vi "CloseConnection.vi"(8 "error in (no error)":errorcluster, 11 "TCP Connection in":refnum<class "TCP Connection.lvclass">) -> (0 "error out":errorcluster, 3 "TCP Connection out":refnum<class "TCP Connection.lvclass">)   [LabVIEW 2011, in "TCP Connection.lvclass"]
doc: "Close a TCP connection.\n\nAuthor: Jared Kirschner"
uses:
  TCP Connection.lvclass
  TCP Connection.lvclass/TCP Connection.ctl
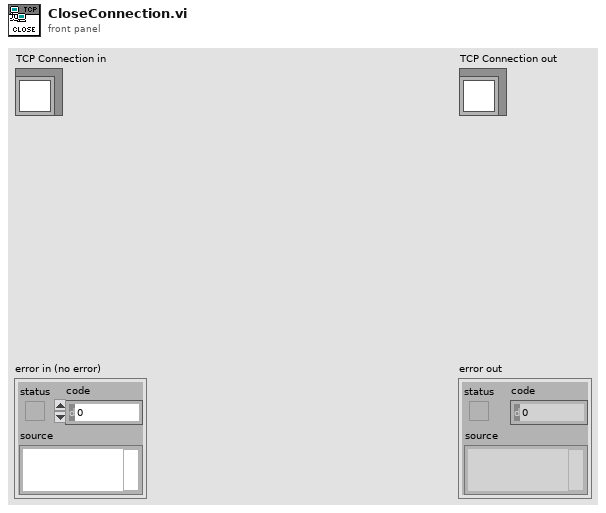
[diagram p1: front panel]
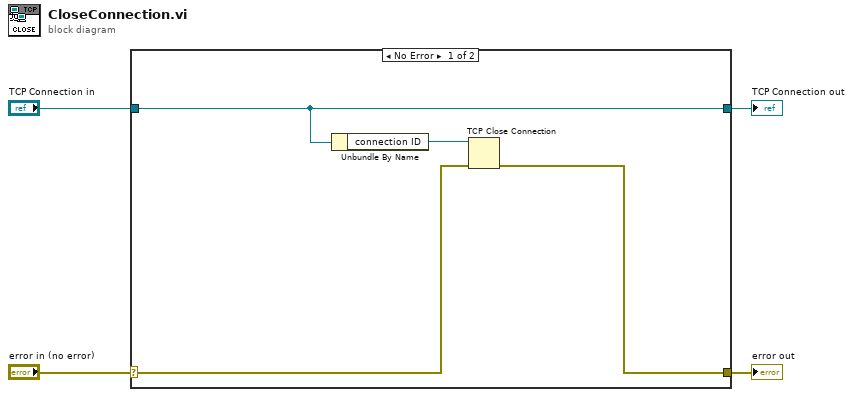
[diagram p0: block diagram]
diagram:
  n1 = case shown="No Error" "error in (no error)" {
    selector: "error in (no error)" -> [w6 w10]
    tunnel: [w5 w10] -> w3
    tunnel: [w8 w9] -> w1
    tunnel: "TCP Connection in" -> [w8 w9]
    frame No Error {
      n2 = Unbundle By Name(w8) -> ("connection ID"=w7:refnum<k5>)
      n3 = TCP Close Connection(connection ID=w7, error in (no error)=w6) -> (error out=w5:errorcluster)  [unwired: 1 in, 1 out]
    }
    frame Error {
    }
  }
  "error out" <- w3
  "TCP Connection out" <- w1
